vi "rqcAlice SyncDetector Control (Low Level Example).vi"() -> ()   [LabVIEW 2019]
uses:
  <vilib>/FPGAPlugInAG/PCI-7811R/niLvFpga_Open_PCI-7811R.vi
  <vilib>/rvi/interface/common/dynamic/niFpgaDynamicAddResources.vi
  <vilib>/FPGAPlugInAG/Dynamic/niLvFpga_Close_Dynamic.vi
  <vilib>/rvi/interface/nirviOpenFPGA/nirviOpenFPGA.xnode
  FPGA Bitfiles/rqcAlice FPGA (7811R) v 3.2.0.lvbitx
  <vilib>/rvi/interface/nirviCloseFPGA/nirviCloseFPGA.xnode
panel:
  in  "send":bool
  in  "Comparator level, V":dbl=1.15 format="%#_13g"
  in  "Offset, V":dbl=1.15 format="%#_13g"
  in  "stop":bool
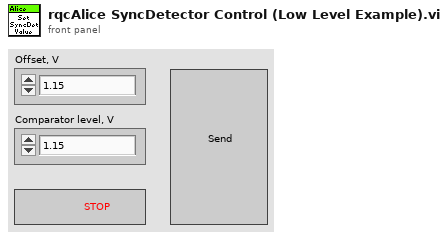
[diagram p1: front panel]
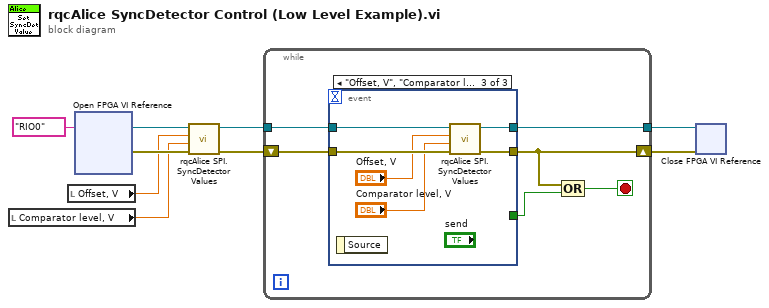
[diagram p0: block diagram]
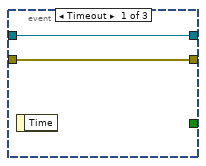
[diagram p2: hidden frame]
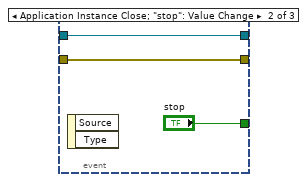
[diagram p3: hidden frame]
diagram:
  n1 = local read "Comparator level, V"() -> (w1:dbl)
  n2 = local read "Offset, V"() -> (w2:dbl)
  n3 = xnode "Open FPGA VI Reference"("resource name"=tag "RIO0") -> ("FPGA VI Reference Out"=w8:refnum<k20>, "error out"=w6:errorcluster)  [unwired: 1 in]
  n4 = call "rqcAlice SPI.SyncDetector Values.vi"("error in"=w6, "Comparator level"=w1, "Offset"=w2, "Alice FPGA Reference In"=w8) -> ("error out"=w5:errorcluster, "Alice FPGA Reference Out"=w7:refnum<k20>)  [unwired: 6 in]
  n5 = while {
    shift-right: [w11] -> w4
    shift-left: w5 -> [w14]
    tunnel: w7 -> [w15]
    tunnel: [w13] -> w3
    stop <- w12 stop-if-true
    n6 = event shown="[2] \"Offset, V\", \"Comparator level, V\", \"send\": Value Change" {
      selector: _ -> [_ _ _]
      dyn-events: _ -> [_ _ _]
      timeout: _ -> [_ _ _]
      tunnel: w15 -> [w16 w19 w26]
      tunnel: w14 -> [w17 w18 w25]
      tunnel: [w17 w18 w24] -> w11
      tunnel: [w16 w19 w23] -> w13
      tunnel: [_ "stop" _] -> w10
      event Timeout {
        n7 = event-data() -> ()  [unwired: 1 in, 1 out]
      }
      event Application Instance Close; "stop": Value Change {
        n8 = event-data() -> ()  [unwired: 1 in, 2 out]
      }
      event "Offset, V", "Comparator level, V", "send": Value Change {
        n9 = event-data() -> ()  [unwired: 1 in, 1 out]
        n10 = call "rqcAlice SPI.SyncDetector Values.vi"("error in"=w25, "Comparator level"="Comparator level, V", "Offset"="Offset, V", "Alice FPGA Reference In"=w26) -> ("error out"=w24:errorcluster, "Alice FPGA Reference Out"=w23:refnum<k20>)  [unwired: 6 in]
      }
    }
    n11 = Compound Arithmetic op=OR(w11, w10) -> (w12:bool)
  }
  n12 = xnode "Close FPGA VI Reference"("FPGA VI Reference In"=w3, "error in"=w4) -> ()  [unwired: 1 out]
